vi "GET IDX VALUE.vi"() -> (3 "Identifier Out":string)   [LabVIEW 2019]
uses:
  <vilib>/addons/database/Auxilliary.llb/DB Tools Cursor Type.ctl
  <vilib>/addons/database/Connection.llb/DB Tools Open Connec (String).vi
  <vilib>/addons/database/Connection.llb/Conn Execute.vi
  <vilib>/addons/database/Recordset.llb/Rec Fetch Recordset Data (R).vi
  <vilib>/addons/database/Recordset.llb/Rec Destroy - Connection.vi
  <vilib>/addons/database/_DB Variant To Data/Database Variant To Data.xnode
  <vilib>/addons/database/NI_Database_API.lvlib
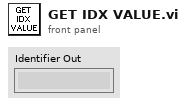
[diagram p1: front panel]
types:
  T1 = typedef "NI_Database_API.lvlib/DB Tools Cursor Type.ctl" = enum16{"forward-only", "keyset", "dynamic", "static"}
  T2 = typedef "NI_Database_API.lvlib/Conn ObjectReference.ctl" = refnum<k1>
  T3 = typedef "NI_Database_API.lvlib/Rec ObjectReference.ctl" = refnum<k1>
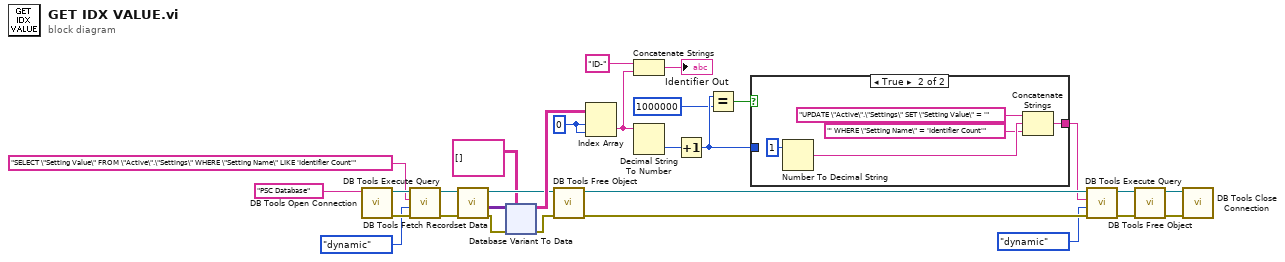
[diagram p0: block diagram]
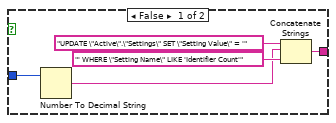
[diagram p2: hidden frame]
diagram:
  w16 = 0 ("index")
  n1 = call-poly <vilib>:"DB Tools Open Connection.vi"("connection information"="PSC Database") -> ("error out"=w27:errorcluster, "connection reference"=w28:T2)  [unwired: 7 in]
  n2 = call-poly <vilib>:"DB Tools Execute Query.vi"("error in (no error)"=w27, "cursor type"=DB_Tools_Cursor_Type."dynamic", "SQL query"="SELECT \"Setting Value\" FROM \"Active\".\"Settings\" WHERE \"Setting Name\" LIKE 'Identifier Count'", "connection reference"=w28) -> ("error out"=w23:errorcluster, "recordset reference"=w24:T3)  [unwired: 4 in]
  n3 = call-poly <vilib>:"DB Tools Fetch Recordset Data.vi"("error in (no error)"=w23, "recordset reference"=w24) -> ("error out"=w21:errorcluster, "recordset data"=w22:variant[][], "recordset reference out"=w19:T3)  [unwired: 3 in]
  n4 = xnode "Database Variant To Data"("database variant"=w22, "error in (no error)"=w21, "type"=string[][] []) -> ("data"=w20:string[][], "error out"=w18:errorcluster)
  n5 = call-poly <vilib>:"DB Tools Free Object.vi"("error in (no error)"=w18, "recordset reference"=w19) -> ("error out"=w7:errorcluster, "connection reference"=w8:T2)  [unwired: 8 in]
  n6 = Index Array(array=w20, index (row)=w16, index (col)=w16) -> (element=w13:string)
  n7 = Concatenate Strings("ID-" ("string"), w13) -> (→"Identifier Out":string)
  n8 = Decimal String To Number(string=w13) -> (number=w15:i32)  [unwired: 2 in, 1 out]
  n9 = Increment(x=w15) -> (x+1=w11:i32)
  n10 = Equal?(x=w11, y=1000000) -> (x = y?=w12:bool)
  n11 = case shown="True" w12 {
    tunnel: w11 -> [w34 _]
    tunnel: [w30 w35] -> w6
    frame False {
      n12 = Number To Decimal String(number=w34) -> (decimal integer string=w31:string)  [unwired: 1 in]
      n13 = Concatenate Strings("UPDATE \"Active\".\"Settings\" SET \"Setting Value\" = '" ("SQL query"), w31, "' WHERE \"Setting Name\" LIKE 'Identifier Count'" ("string")) -> (w30:string)
    }
    frame True {
      n14 = Number To Decimal String(number=1) -> (decimal integer string=w37:string)  [unwired: 1 in]
      n15 = Concatenate Strings("UPDATE \"Active\".\"Settings\" SET \"Setting Value\" = '" ("SQL query"), w37, "' WHERE \"Setting Name\" = 'Identifier Count'" ("string")) -> (w35:string)
    }
  }
  n16 = call-poly <vilib>:"DB Tools Execute Query.vi"("error in (no error)"=w7, "cursor type"=DB_Tools_Cursor_Type."dynamic", "SQL query"=w6, "connection reference"=w8) -> ("error out"=w3:errorcluster, "recordset reference"=w4:T3)  [unwired: 4 in]
  n17 = call-poly <vilib>:"DB Tools Free Object.vi"("error in (no error)"=w3, "recordset reference"=w4) -> ("error out"=w1:errorcluster, "connection reference"=w2:T2)  [unwired: 8 in]
  n18 = call <vilib>:"DB Tools Close Connection.vi"("error in (no error)"=w1, "connection reference"=w2) -> ()  [unwired: 5 in, 1 out]
